vi "lvEtherbone.device_close.vi"(0 "eb_socket_ID":i32, 1 "eb_device_ID":i32, 5 "error in (no error)":errorcluster) -> (13 "eb_status":T1 items=["EB_SUCCESS"=1, "EB_OK"=0, "EB_FAIL"=-1, "EB_ADDRESS"=-2, "EB_WIDTH"=-3, "EB_OVERFLOW"=-4, "EB_ENDIAN"=-5, "EB_BUSY"=-6, "EB_TIMEOUT"=-7, "EB_OOM"=-8, "EB_ABI"=-9, "EB_SEGFAULT"=-10], 14 "eb_socket_ID out":i32, 19 "error out":errorcluster)   [LabVIEW 2012, in "lvEtherbone.lvlib"]
doc: "/* Close a remote Etherbone device.\n * Any inflight or ready-to-send cycles will receive EB_TIMEOUT.\n *\n * Return codes:\n * OK - associated memory has been freed\n * BUSY - there are unclosed wishbone cycles on this device\n */\nEB_PUBLIC\neb_status_t eb_device_close(eb_device_t device);"
uses:
  lvEtherbone.lvlib
  lvEtherbone.lveb_status_t.ctl
  libetherbone.so
panel:
  in  "eb_status_t":T1 items=["EB_SUCCESS"=1, "EB_OK"=0, "EB_FAIL"=-1, "EB_ADDRESS"=-2, "EB_WIDTH"=-3, "EB_OVERFLOW"=-4, "EB_ENDIAN"=-5, "EB_BUSY"=-6, "EB_TIMEOUT"=-7, "EB_OOM"=-8, "EB_ABI"=-9, "EB_SEGFAULT"=-10]
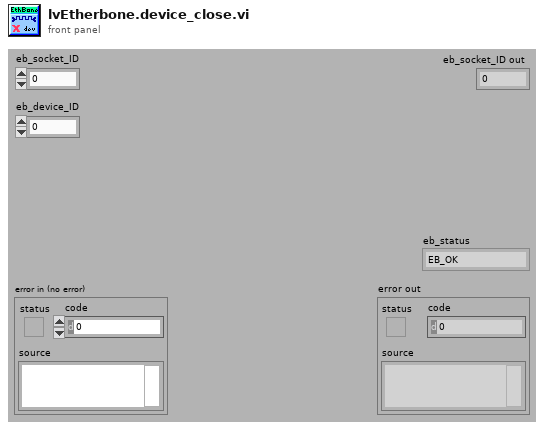
[diagram p1: front panel]
types:
  T1 = typedef "lvEtherbone.lvlib/lvEtherbone.lveb_status_t.ctl" = i32
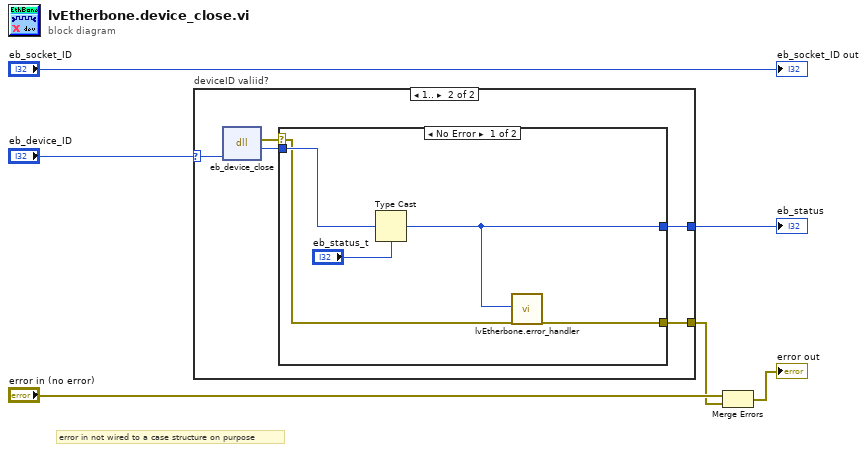
[diagram p0: block diagram]
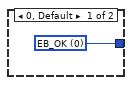
[diagram p2: hidden frame]
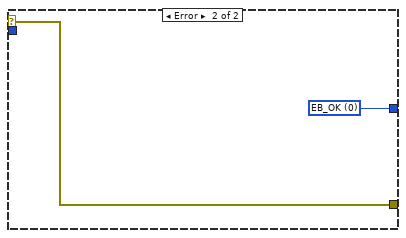
[diagram p3: hidden frame]
diagram:
  # "error in not wired to a case structure on purpose"
  n1 = case "deviceID valiid?" shown="1.." "eb_device_ID" {
    selector: "eb_device_ID" -> [_ w8]
    tunnel: [w7 w12] -> w6
    tunnel: [_ w9] -> w4
    frame 0, Default {
      w7 = T1 0 items=["EB_SUCCESS"=1, "EB_OK"=0, "EB_FAIL"=-1, "EB_ADDRESS"=-2, "EB_WIDTH"=-3, "EB_OVERFLOW"=-4, "EB_ENDIAN"=-5, "EB_BUSY"=-6, "EB_TIMEOUT"=-7, "EB_OOM"=-8, "EB_ABI"=-9, "EB_SEGFAULT"=-10] ("eb_status_t")
    }
    frame 1.. {
      n2 = dll-call lib="libetherbone.so" fn="eb_device_close"("eb_device_ID"=w8) -> (error out=w10:errorcluster, "eb_status"=w11:i32)  [unwired: 4 in, 1 out]
      n3 = case shown="No Error" w10 {
        selector: w10 -> [w13 w19]
        tunnel: w11 -> [w17 _]
        tunnel: [w15 w18] -> w12
        tunnel: [w14 w19] -> w9
        frame No Error {
          n4 = Type Cast(type="eb_status_t", x=w17) -> (*(type *) &x=w15:T1)
          n5 = call "lvEtherbone.error_handler.vi"("eb_status"=w15, "error in"=w13) -> ("error out"=w14:errorcluster)  [unwired: 17 in]
        }
        frame Error {
          w18 = T1 0 items=["EB_SUCCESS"=1, "EB_OK"=0, "EB_FAIL"=-1, "EB_ADDRESS"=-2, "EB_WIDTH"=-3, "EB_OVERFLOW"=-4, "EB_ENDIAN"=-5, "EB_BUSY"=-6, "EB_TIMEOUT"=-7, "EB_OOM"=-8, "EB_ABI"=-9, "EB_SEGFAULT"=-10] ("eb_status_t")
        }
      }
    }
  }
  "eb_status" <- w6
  n6 = Merge Errors("error in (no error)", w4) -> (→"error out":errorcluster)
  "eb_socket_ID out" <- "eb_socket_ID"
